vi "Kowariancja i wsp korelacji.vi"(9 "Wyjscie":dbl[](array[numeric]), 10 "Liczba probek":i32, 11 "Wyjscie 2":dbl[](array[numeric])) -> (2 "Korelacja":dbl, 3 "Kowariancja":dbl)   [LabVIEW 2019]
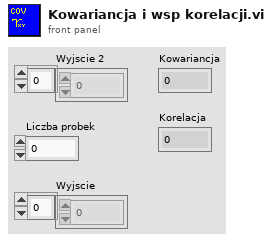
[diagram p1: front panel]
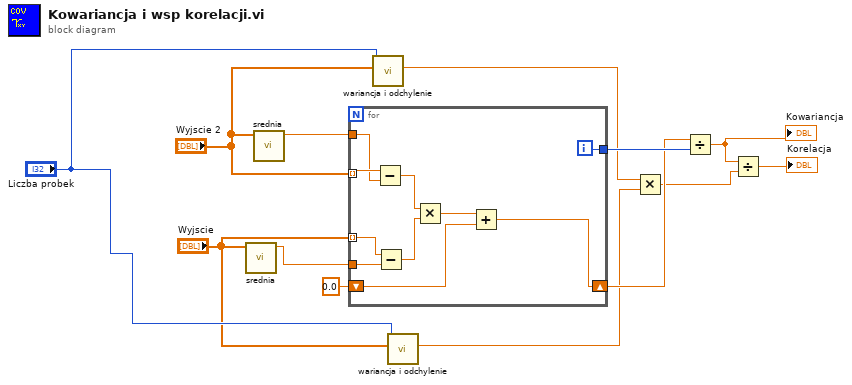
[diagram p0: block diagram]
diagram:
  n1 = call "srednia.vi"("Array"="Wyjscie") -> ("Srednia"=w2:dbl)  [unwired: 8 in, 2 out]
  n2 = call "srednia.vi"("Array"="Wyjscie 2") -> ("Srednia"=w1:dbl)  [unwired: 8 in, 2 out]
  n3 = for {
    tunnel: "Wyjscie 2" -> [w23] mode=indexing
    tunnel: w1 -> [w22]
    tunnel: "Wyjscie" -> [w21] mode=indexing
    tunnel: w2 -> [w20]
    shift-right: [w15] -> w12
    shift-left: 0.0 -> [w16]
    tunnel: [w14] -> w13
    i -> [w14]
    n4 = Subtract(x=w23, y=w22) -> (x-y=w18:dbl)
    n5 = Subtract(x=w21, y=w20) -> (x-y=w19:dbl)
    n6 = Multiply(x=w18, y=w19) -> (x*y=w17:dbl)
    n7 = Add(x=w17, y=w16) -> (x+y=w15:dbl)
  }
  n8 = call "wariancja i odchylenie.vi"("Array"="Wyjscie 2", "Liczba probek"="Liczba probek") -> ("Odchylenie\nstandardowe"=w7:dbl)  [unwired: 8 in, 1 out]
  n9 = call "wariancja i odchylenie.vi"("Array"="Wyjscie", "Liczba probek"="Liczba probek") -> ("Odchylenie\nstandardowe"=w8:dbl)  [unwired: 8 in, 1 out]
  n10 = Multiply(x=w7, y=w8) -> (x*y=w9:dbl)
  n11 = Divide(x=w12, y=w13) -> (x/y=w11:dbl)
  "Kowariancja" <- w11
  n12 = Divide(x=w11, y=w9) -> (x/y=→"Korelacja":dbl)
